vi "Set Module Ref.vi"(8 "error in (no error)":errorcluster, 11 "Core in":refnum<class "Core.lvclass">) -> (0 "error out":errorcluster, 3 "Core out":refnum<class "Core.lvclass">)   [LabVIEW 2019]
uses:
  Core.lvclass
  ModuleAbstract/ModuleAbstract.lvclass
  C:/Projekty/_Wewnetrzne/PC_ActorFramework/07_Program/LABVIEW/02_Source/Modules/ModuleAbstract/ModuleAbstract.lvclass
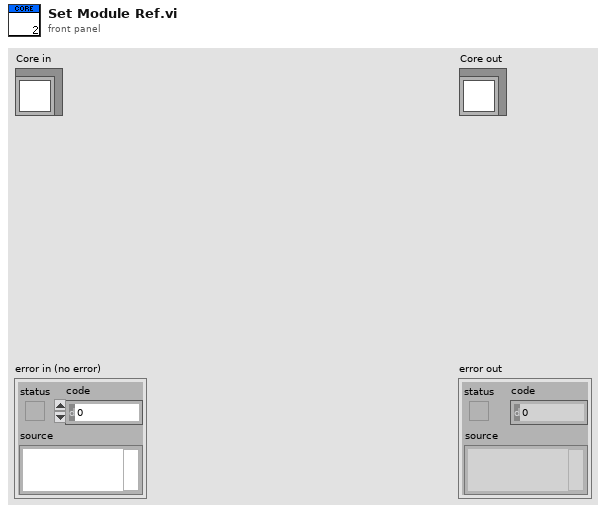
[diagram p1: front panel]
types:
  T1 = cluster{"Core":cluster{"ModuleRef":refnum<class "Message Enqueuer.lvclass">, "UIRef":refnum<class "Message Enqueuer.lvclass">}, "MainPanel":cluster{"ModuleRef":refnum<class "Message Enqueuer.lvclass">, "UIRef":refnum<class "Message Enqueuer.lvclass">}, "UserManagment":cluster{"ModuleRef":refnum<class "Message Enqueuer.lvclass">, "UIRef":refnum<class "Message Enqueuer.lvclass">}, "Hardware":cluster{"ModuleRef":refnum<class "Message Enqueuer.lvclass">, "UIRef":refnum<class "Message Enqueuer.lvclass">}, "Systems":cluster{"ModuleRef":refnum<class "Message Enqueuer.lvclass">, "UIRef":refnum<class "Message Enqueuer.lvclass">}, "DataAcq":cluster{"ModuleRef":refnum<class "Message Enqueuer.lvclass">, "UIRef":refnum<class "Message Enqueuer.lvclass">}, "Steering":cluster{"ModuleRef":refnum<class "Message Enqueuer.lvclass">, "UIRef":refnum<class "Message Enqueuer.lvclass">}, "DataProcessing":cluster{"ModuleRef":refnum<class "Message Enqueuer.lvclass">, "UIRef":refnum<class "Message Enqueuer.lvclass">}}
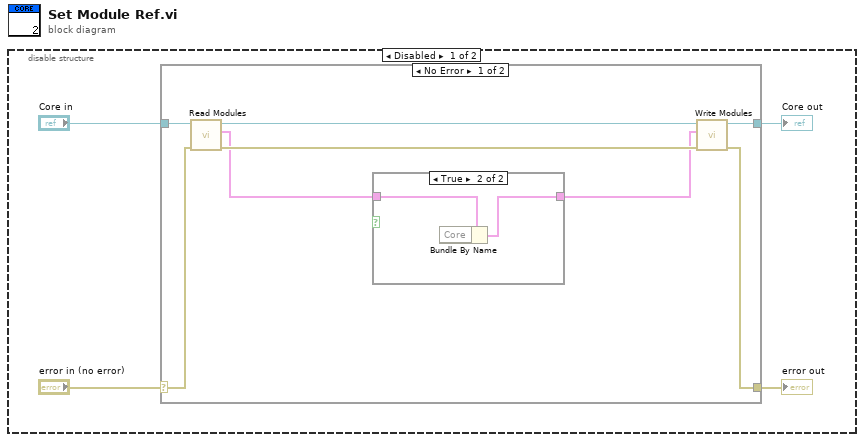
[diagram p0: block diagram]
diagram:
  n1 = disable-structure shown="Disabled" {
    frame Disabled {
      n2 = case shown="No Error" "error in (no error)" {
        selector: "error in (no error)" -> [w9 w16]
        tunnel: [w7 w16] -> w3
        tunnel: [w10 w15] -> w1
        tunnel: "Core in" -> [w12 w15]
        frame No Error {
          n3 = call "Read Modules.vi"("error in (no error)"=w9, "ModuleAbstract in"=w12) -> ("error out"=w8:errorcluster, "Modules"=w6:T1, "ModuleAbstract out"=w11:refnum<class "Core.lvclass">)  [unwired: 7 in]
          n4 = case shown="True" {
            selector: _ -> [_ _]
            tunnel: w6 -> [_ w14]
            tunnel: [_ w13] -> w5
            frame False {
            }
            frame True {
              n5 = Bundle By Name(cluster=w14) -> (w13:T1)  [unwired: 1 in]
            }
          }
          n6 = call "Write Modules.vi"("error in (no error)"=w8, "Modules"=w5, "ModuleAbstract in"=w11) -> ("error out"=w7:errorcluster, "ModuleAbstract out"=w10:refnum<class "Core.lvclass">)  [unwired: 7 in]
        }
        frame Error {
        }
      }
      "error out" <- w3
      "Core out" <- w1
    }
    frame Enabled {
    }
  }
